vi "GetFaultListBatt_rack.vi"(1 "Warn":u16 format="%x", 2 "Err2":u16 format="%x", 3 "Err1":u16 format="%x") -> (0 "Error/Warning list":string)   [LabVIEW 2021]
panel:
  in  "Warn string":string[](array[string])=["", "Reduced power to prevent overvoltage", "Reduced power to prevent undervoltage", "Reduced power due to undertemperature", "Reduced power due to overertemperature", "", "", "", "", "Yellow flag", "Watchdog disabled", "", "", "", "", ""]
  in  "Err2 string":string[](array[string])=["Roof fan error", "Isolation error", "Emergency button", "Yellow flag timeout", "Watchdog error", "", "", "", "", "", "", "", "", "", "", "Other Errors"]
  in  "Err1 string":string[](array[string])=["OverCurrent", "OvervVoltage", "UnderVoltage", "UnderTemperature", "OverTemperature", "SelfTest Error", "DC-power cable missing", "External stop from I/O", "Incompatible SRB modules in string", "Fan error (SRB)", "Broken wire detected", "Communication error current sensor", "Communication error second level safety", "Thirs level safety error", "Contactor error", "Service Necessary"]
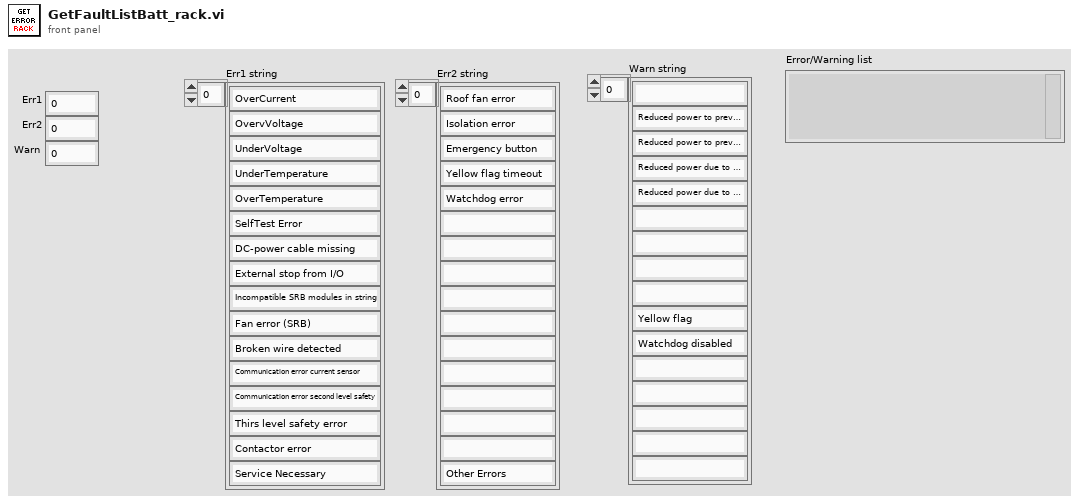
[diagram p1: front panel]
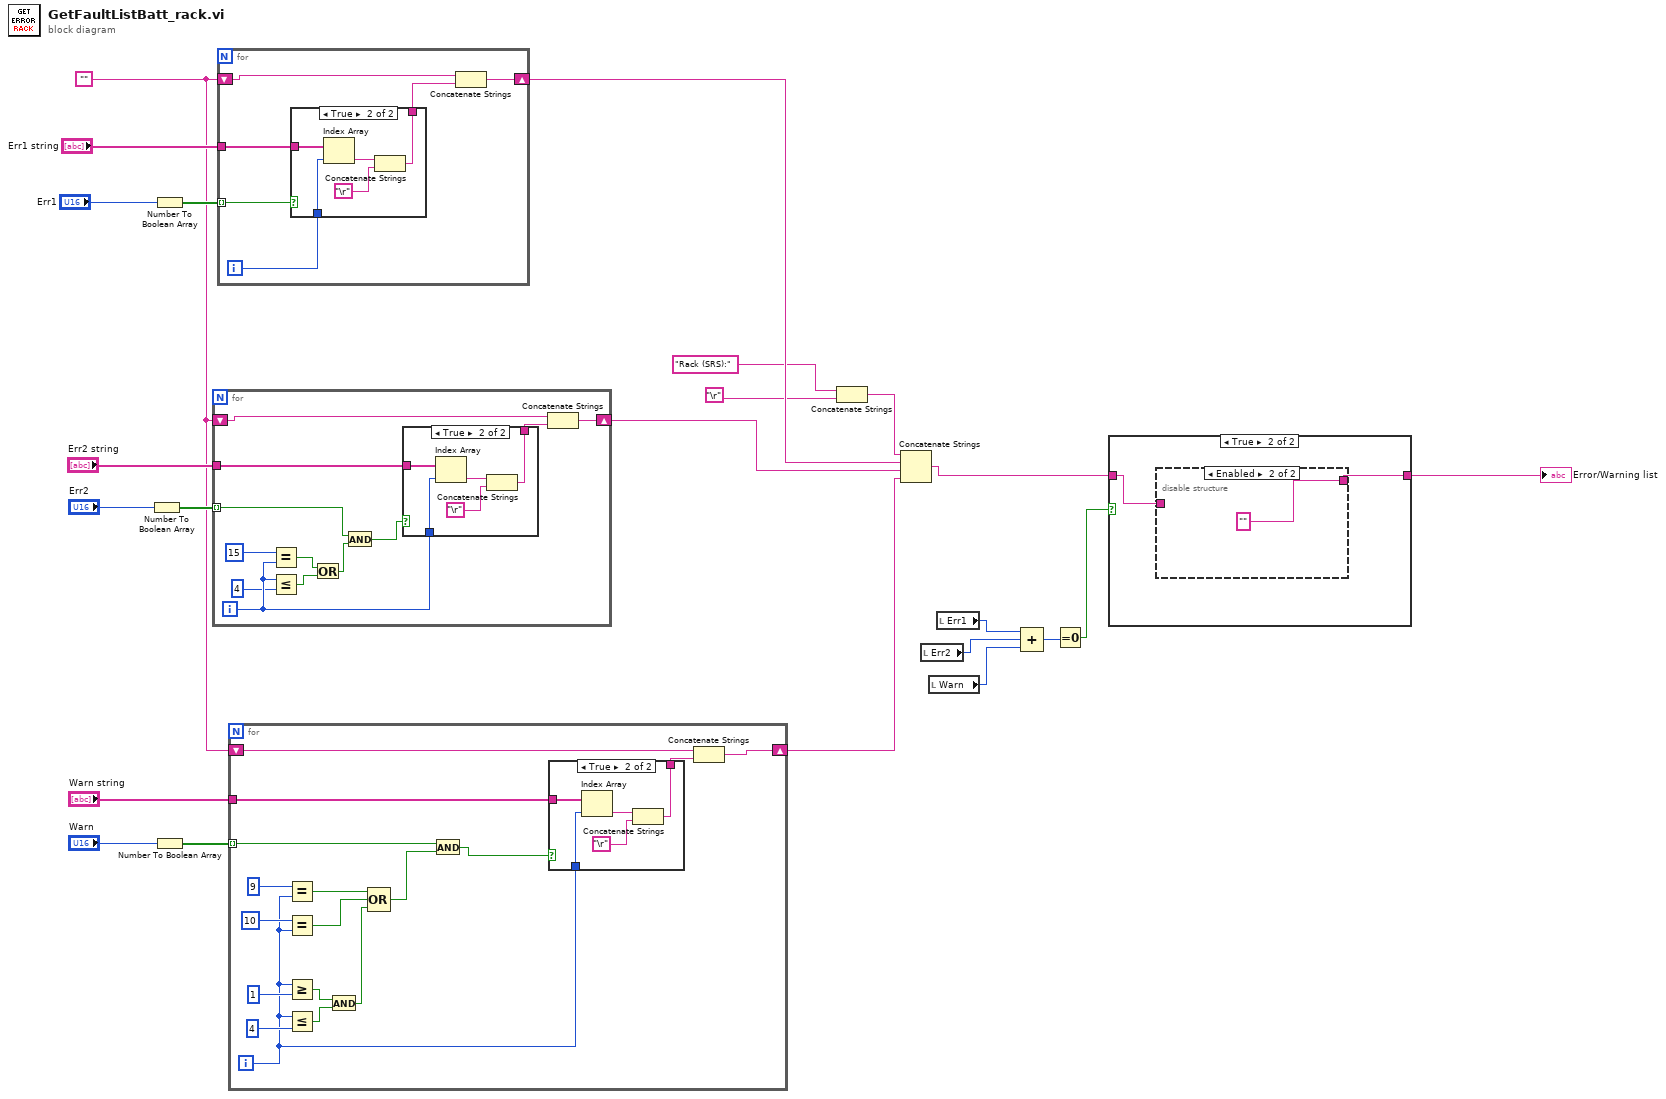
[diagram p0: block diagram]
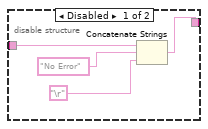
[diagram p3: hidden frame]
diagram:
  w13 = ""
  n1 = Number To Boolean Array(number="Err2") -> (Boolean array=w18:bool[])
  n2 = Number To Boolean Array(number="Err1") -> (Boolean array=w21:bool[])
  n3 = Number To Boolean Array(number="Warn") -> (Boolean array=w10:bool[])
  n4 = for {
    shift-right: [w34] -> w16
    shift-left: w13 -> [w35]
    tunnel: "Err2 string" -> [w29]
    tunnel: w18 -> [w27] mode=indexing
    i -> [w25]
    n5 = Equal?(x=15, y=w25) -> (x = y?=w30:bool)
    n6 = Less Or Equal?(x=w25, y=4 ("x")) -> (x <= y?=w31:bool)
    n7 = Or(x=w30, y=w31) -> (x .or. y?=w28:bool)
    n8 = And(x=w27, y=w28) -> (x .and. y?=w26:bool)
    n9 = case shown="True" w26 {
      tunnel: w29 -> [_ w37]
      tunnel: w25 -> [_ w40]
      tunnel: [_ w38] -> w33
      frame False {
      }
      frame True {
        n10 = Index Array(array=w37, index=w40) -> (element=w36:string)
        n11 = Concatenate Strings(w36, "\r") -> (w38:string)
      }
    }
    n12 = Concatenate Strings(w35, w33) -> (w34:string)
  }
  n13 = for {
    tunnel: "Err1 string" -> [w46]
    tunnel: w21 -> [w45] mode=indexing
    shift-right: [w43] -> w17
    shift-left: w13 -> [w44]
    i -> [w41]
    n14 = case shown="True" w45 {
      tunnel: w46 -> [_ w48]
      tunnel: w41 -> [_ w51]
      tunnel: [_ w49] -> w42
      frame False {
      }
      frame True {
        n15 = Index Array(array=w48, index=w51) -> (element=w47:string)
        n16 = Concatenate Strings(w47, "\r") -> (w49:string)
      }
    }
    n17 = Concatenate Strings(w44, w42) -> (w43:string)
  }
  n18 = for {
    shift-right: [w67] -> w9
    shift-left: w13 -> [w68]
    tunnel: "Warn string" -> [w64]
    tunnel: w10 -> [w58] mode=indexing
    i -> [w52]
    n19 = Equal?(x=9, y=w52) -> (x = y?=w62:bool)
    n20 = Equal?(x=10, y=w52) -> (x = y?=w61:bool)
    n21 = Greater Or Equal?(x=w52, y=1 ("x")) -> (x >= y?=w56:bool)
    n22 = Less Or Equal?(x=w52, y=4 ("x")) -> (x <= y?=w55:bool)
    n23 = And(x=w56, y=w55) -> (x .and. y?=w57:bool)
    n24 = Compound Arithmetic op=OR(w62, w61, w57) -> (w60:bool)
    n25 = And(x=w58, y=w60) -> (x .and. y?=w59:bool)
    n26 = case shown="True" w59 {
      tunnel: w64 -> [_ w70]
      tunnel: w52 -> [_ w73]
      tunnel: [_ w71] -> w66
      frame False {
      }
      frame True {
        n27 = Index Array(array=w70, index=w73) -> (element=w69:string)
        n28 = Concatenate Strings(w69, "\r") -> (w71:string)
      }
    }
    n29 = Concatenate Strings(w68, w66) -> (w67:string)
  }
  n30 = Concatenate Strings("Rack (SRS):" ("string"), "\r") -> (w3:string)
  n31 = Concatenate Strings(w3, w17, w16, w9) -> (w1:string)
  n32 = local read "Err2"() -> (w7:u16)
  n33 = local read "Warn"() -> (w6:u16)
  n34 = local read "Err1"() -> (w8:u16)
  n35 = Compound Arithmetic op=ADD(w8, w7, w6) -> (w5:u16)
  n36 = Equal To 0?(x=w5) -> (x = 0?=w4:bool)
  n37 = case shown="True" w4 {
    tunnel: [w74 w76] -> w2
    tunnel: w1 -> [w74 w75]
    frame False {
    }
    frame True {
      n38 = disable-structure shown="Enabled" {
        disable-tunnel: [w80 ""] -> w76
        disable-tunnel: w75 -> [w79 _]
        frame Disabled {
          n39 = Concatenate Strings(w79, "No Error" ("string"), "\r") -> (w80:string)
        }
        frame Enabled {
        }
      }
    }
  }
  "Error/Warning list" <- w2
